vi "FuncImg-Load stack.vi"(1 "RedFile":string="Red*", 2 "GreenFile":string="Green*", 11 "Error In":errorcluster) -> (8 "RedMaxZ":T1, 10 "GreenMaxZ":T1, 14 "Number of Files":i32, 15 "Error Out":errorcluster)   [LabVIEW 2013]
uses:
  <vilib>/vision/Image Controls.llb/IMAQ Image.ctl
  Typedefs/Get-Set-Clear Control.ctl
  <vilib>/vision/NI_Vision_Development_Module.lvlib
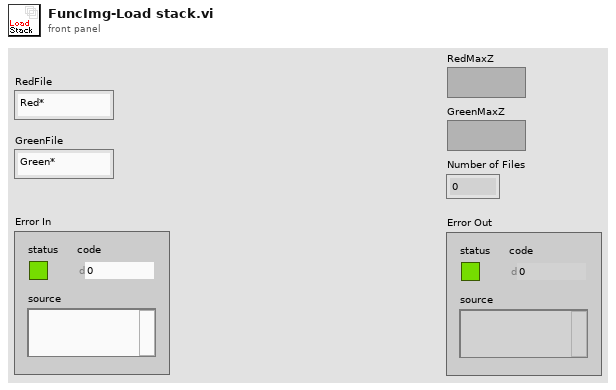
[diagram p1: front panel]
types:
  T1 = typedef "IMAQ Image.ctl" = refnum<image>
  T2 = typedef "Get-Set-Clear Control.ctl" = enum16{"Get", "Set", "Clear"}
  T3 = enum32{"Average", "Min", "Max", "Clear  if < ", "Clear  if < or =", "Clear  if =", "Clear  if > or =", "Clear  if >"}
  T4 = typedef "Image Type" = u32
  T5 = typedef "Fixed strings.ctl" = cluster{"ROI file name":string, "Normalised ROI file name":string, "Zplane Pockels values file name":string, "Functional data folder name":string, "Experiment Header file name":string, "Z-stack images folder name":string, "Groups setup rel. path":string, "Groups text file rel. path":string, "TDMS files folder name (F.img)":string, "TDMS files folder name (V.acq)":string, "TDMS files folder name (Pl.acq)":string, "Cycle rel times sequence file":string, "Dynamically called VIs folder name":string, "Time Series folder base name":string}
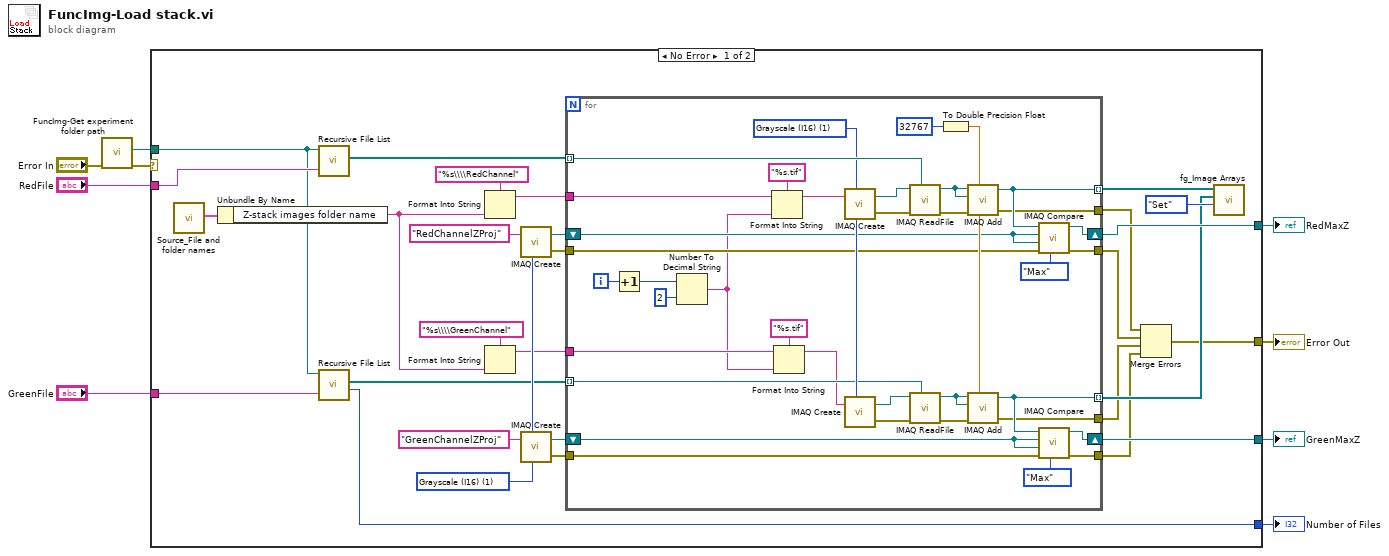
[diagram p0: block diagram]
diagram:
  n1 = call "FuncImg-Get experiment folder path.vi"("error in (no error)"="Error In") -> ("error out"=w2:errorcluster, "Experiment data folder path"=w1:path)  [unwired: 9 in]
  n2 = case shown="No Error" w2 {
    selector: w2 -> [_ w76]
    tunnel: [w31 _] -> w9
    tunnel: [w30 _] -> w8
    tunnel: [w29 _] -> w7
    tunnel: "RedFile" -> [w27 _]
    tunnel: "GreenFile" -> [w25 _]
    tunnel: [w19 w76] -> w4
    tunnel: w1 -> [w10 _]
    frame No Error {
      w38 = T4 1 items=["Grayscale (U8)", "Grayscale (I16)", "Grayscale (SGL)", "Complex (CSG)", "RGB (U32)", "HSL (U32)", "RGB (U64)"] ("Image Type")
      n3 = call "Source_File and folder names.vi"() -> ("Fixed strings"=w11:T5)  [unwired: 1 in]
      n4 = Unbundle By Name(w11) -> ("Z-stack images folder name"=w12:string)
      n5 = call <vilib>:"Recursive File List.vi"("pattern"=w27, "Folder Path"=w10) -> ("All Files in Dir"=w26:path[])  [unwired: 5 in, 4 out]
      n6 = call <vilib>:"Recursive File List.vi"("pattern"=w25, "Folder Path"=w10) -> ("Number of Files"=w29:i32, "All Files in Dir"=w28:path[])  [unwired: 5 in, 3 out]
      n7 = Format Into String(format string="%s\\\\RedChannel", w12) -> (resulting string=w14:string)  [unwired: 2 in, 1 out]
      n8 = Format Into String(format string="%s\\\\GreenChannel", w12) -> (resulting string=w13:string)  [unwired: 2 in, 1 out]
      n9 = call "IMAQ Create"("Image Name"="RedChannelZProj" ("string"), "Image Type"=w38) -> ("New Image"=w33:T1, "error out"=w32:errorcluster)  [unwired: 3 in]
      n10 = call "IMAQ Create"("Image Name"="GreenChannelZProj" ("string"), "Image Type"=w38) -> ("New Image"=w35:T1, "error out"=w34:errorcluster)  [unwired: 3 in]
      n11 = for {
        tunnel: [w59] -> w23 mode=indexing
        tunnel: [w60] -> w22 mode=indexing
        tunnel: w28 -> [w48] mode=indexing
        tunnel: [w54] -> w21
        tunnel: [w52] -> w18
        shift-right: [w70] -> w31
        shift-left: w35 -> [w51]
        tunnel: [w69] -> w17
        tunnel: w34 -> [w68]
        shift-right: [w67] -> w30
        shift-left: w33 -> [w46]
        tunnel: w32 -> [w47]
        tunnel: [w66] -> w20
        tunnel: w26 -> [w57] mode=indexing
        tunnel: w14 -> [w45]
        tunnel: w13 -> [w41]
        i -> [w56]
        w50 = T4 1 items=["Grayscale (U8)", "Grayscale (I16)", "Grayscale (SGL)", "Complex (CSG)", "RGB (U32)", "HSL (U32)", "RGB (U64)"] ("Image Type")
        n12 = Increment(x=w56) -> (x+1=w58:i32)
        n13 = Number To Decimal String(number=w58, width (-)=i16 2) -> (decimal integer string=w39:string)
        n14 = Format Into String(format string="%s.tif", initial string=w45, w39) -> (resulting string=w43:string)  [unwired: 1 in, 1 out]
        n15 = Format Into String(format string="%s.tif", initial string=w41, w39) -> (resulting string=w40:string)  [unwired: 1 in, 1 out]
        n16 = call "IMAQ Create"("Image Name"=w43, "Image Type"=w50) -> ("New Image"=w74:T1, "error out"=w75:errorcluster)  [unwired: 3 in]
        n17 = call "IMAQ Create"("Image Name"=w40, "Image Type"=w50) -> ("New Image"=w73:T1, "error out"=w72:errorcluster)  [unwired: 3 in]
        n18 = call "IMAQ ReadFile"("File Path"=w57, "error in (no error)"=w75, "Image"=w74) -> ("error out"=w55:errorcluster, "Image Out"=w62:T1)  [unwired: 4 in, 3 out]
        n19 = call "IMAQ ReadFile"("File Path"=w48, "error in (no error)"=w72, "Image"=w73) -> ("error out"=w53:errorcluster, "Image Out"=w63:T1)  [unwired: 4 in, 3 out]
        n20 = To Double Precision Float(number=i16 32767 ("Constant")) -> (double precision float=w49:dbl)
        n21 = call "IMAQ Add"("Image Src A"=w62, "Constant"=w49, "Image Dst"=w62, "error in (no error)"=w55) -> ("Image Dst Out"=w59:T1, "error out"=w54:errorcluster)  [unwired: 3 in]
        n22 = call "IMAQ Add"("Image Src A"=w63, "Constant"=w49, "Image Dst"=w63, "error in (no error)"=w53) -> ("Image Dst Out"=w60:T1, "error out"=w52:errorcluster)  [unwired: 3 in]
        n23 = call "IMAQ Compare"("Operator"=T3."Max", "error in (no error)"=w47, "Image Src B"=w46, "Image Dst"=w46, "Image Src A"=w59) -> ("error out"=w66:errorcluster, "Image Dst Out"=w67:T1)  [unwired: 5 in]
        n24 = call "IMAQ Compare"("Operator"=T3."Max", "error in (no error)"=w68, "Image Src B"=w51, "Image Dst"=w51, "Image Src A"=w60) -> ("error out"=w69:errorcluster, "Image Dst Out"=w70:T1)  [unwired: 5 in]
      }
      n25 = Merge Errors(w21, w20, w18, w17) -> (w19:errorcluster)
      n26 = call "fg_Image Arrays.vi"("Function"=Get-Set-Clear_Control."Set", "Green Images Array in"=w22, "Red Images Array in"=w23) -> ()  [unwired: 7 in, 2 out]
    }
    frame Error {
    }
  }
  "RedMaxZ" <- w8
  "GreenMaxZ" <- w9
  "Number of Files" <- w7
  "Error Out" <- w4
